vi "04_SignalGeneration.vi"() -> ()   [LabVIEW 2019]
uses:
  <vilib>/Analysis/NI_AALBase.lvlib
panel:
  in  "Square":bool
  in  "Triangle":bool
  in  "Sine":bool
  out "Wave":dbl[](graph)
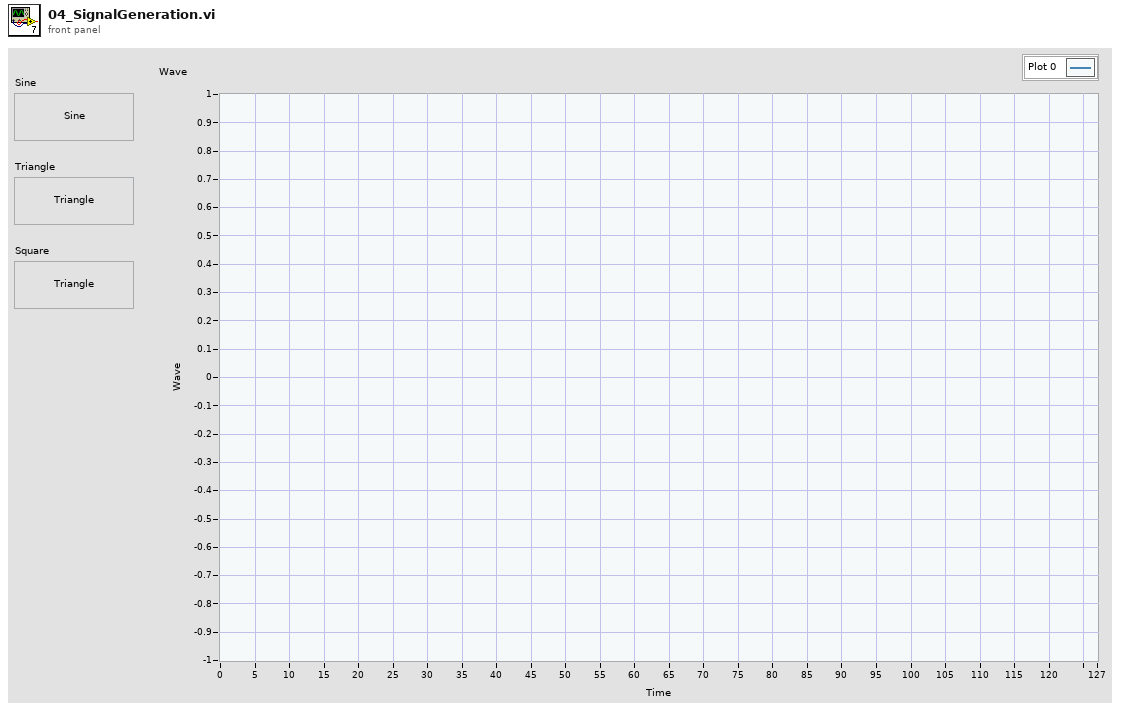
[diagram p1: front panel]
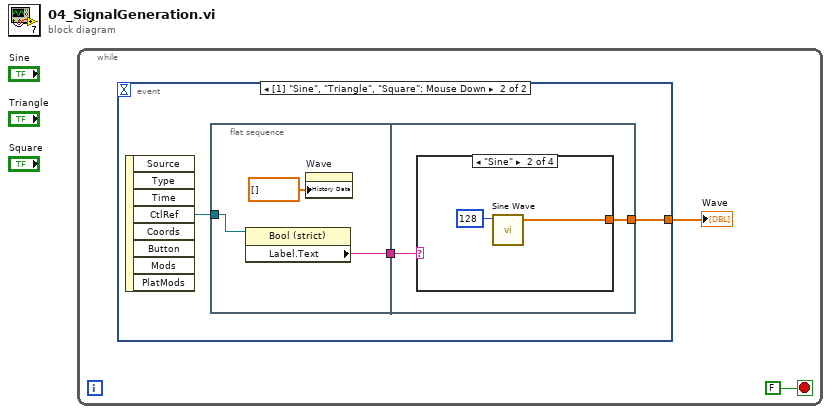
[diagram p0: block diagram]
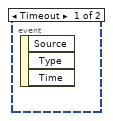
[diagram p2: hidden frame]
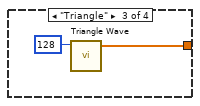
[diagram p4: hidden frame]
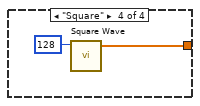
[diagram p5: hidden frame]
diagram:
  n1 = while {
    stop <- FALSE stop-if-true
    n2 = event shown="[1] \"Sine\", \"Triangle\", \"Square\": Mouse Down" {
      selector: _ -> [_ _]
      dyn-events: _ -> [_ _]
      timeout: _ -> [_ _]
      tunnel: [_ w5] -> w2
      event Timeout {
        n3 = event-data() -> ()  [unwired: 1 in, 3 out]
      }
      event "Sine", "Triangle", "Square": Mouse Down {
        n4 = event-data() -> ("CtlRef"=w4:refnum<vi>)  [unwired: 1 in, 7 out]
        n5 = flat-sequence {
          tunnel: w4 -> [w7]
          tunnel: [w6] -> w3
          tunnel: [w10] -> w5
          tunnel: w3 -> [w9]
          frame #0 {
            n6 = property class="Bool (strict)"(reference=w7) -> ("Label.Text"=w6:string)  [unwired: 1 in, 2 out]
            n7 = property on="Wave" class="WFChart (strict)"("History Data"=dbl[] []) -> ()  [unwired: 2 in, 2 out]
          }
          frame #1 {
            n8 = case shown="\"Sine\"" w9 {
              tunnel: [_ w11 w13 w15] -> w10
              frame Default {
              }
              frame "Sine" {
                n9 = call <vilib>:"Sine Wave.vi"("samples"=128) -> ("sine wave"=w11:dbl[])  [unwired: 4 in, 2 out]
              }
              frame "Triangle" {
                n10 = call <vilib>:"Triangle Wave.vi"("samples"=128) -> ("triangle wave"=w13:dbl[])  [unwired: 4 in, 2 out]
              }
              frame "Square" {
                n11 = call <vilib>:"Square Wave.vi"("samples"=128) -> ("square wave"=w15:dbl[])  [unwired: 5 in, 2 out]
              }
            }
          }
        }
      }
    }
    "Wave" <- w2
  }
